vi "Convert_°C_TO_°F.vi"(1 "Temperatura aleatoria °c":dbl, 2 "Temperatura °C":dbl, 3 "Manual/Automatico":bool) -> (0 "Temperatura °F":dbl)   [LabVIEW 2018]
doc: "Esta funcion convierte de grados celcius a grados farenheit. \n\nParametro de entrada: Grados Celcius\nParametro de Salida: Grados Farenheit"
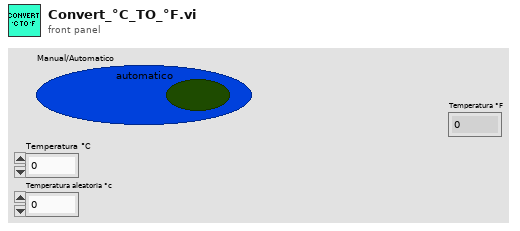
[diagram p1: front panel]
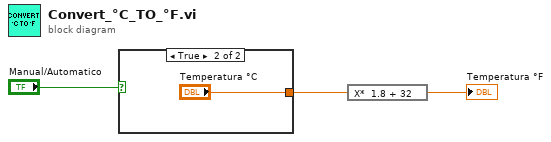
[diagram p0: block diagram]
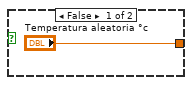
[diagram p2: hidden frame]
diagram:
  n1 = case shown="True" "Manual/Automatico" {
    tunnel: ["Temperatura aleatoria °c" "Temperatura °C"] -> w1
    frame False {
    }
    frame True {
    }
  }
  n2 = expression code="X*  1.8 + 32"(w1) -> (→"Temperatura °F":dbl)
